vi "Initialization.vi"(8 "error in (no error)":errorcluster, 9 "Side":enum16{"Load", "Drive"}(ring), 10 "CtrlRefs":refnum<vi>[](array[refnum]), 11 "TestSinWaveProc in":refnum<class "TestSinWaveProc.lvclass">) -> (0 "error out":errorcluster, 3 "TestSinWaveProc out":refnum<class "TestSinWaveProc.lvclass">)   [LabVIEW 2024, in "TestSinWaveActor.lvlib" / "TestSinWaveProc.lvclass"]
uses:
  TestSinWaveProc.lvclass
  TestSinWaveProc.lvclass/TestSinWaveProc.ctl
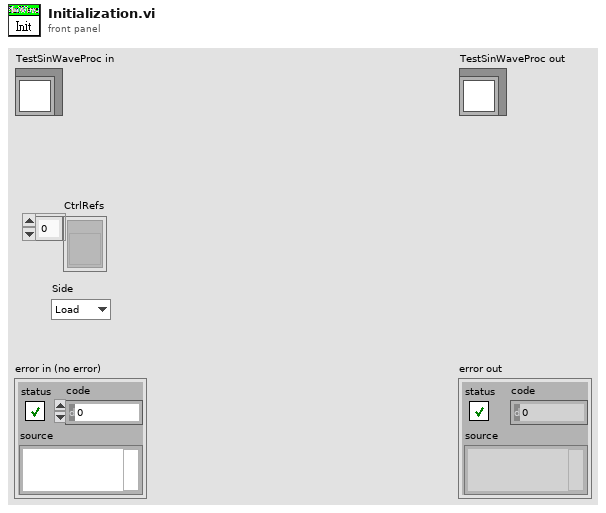
[diagram p1: front panel]
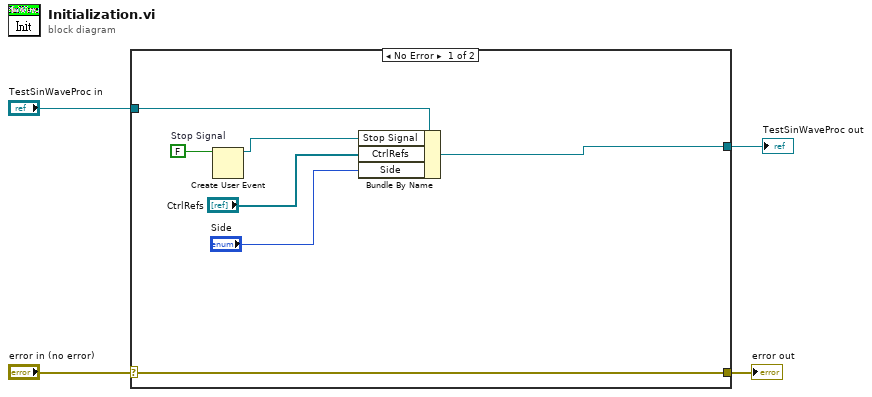
[diagram p0: block diagram]
diagram:
  n1 = case shown="No Error" "error in (no error)" {
    selector: "error in (no error)" -> [w11 w13]
    tunnel: [w11 w13] -> w3
    tunnel: [w6 w12] -> w1
    tunnel: "TestSinWaveProc in" -> [w7 w12]
    frame No Error {
      w10 = FALSE  # Stop Signal
      n2 = Create User Event(user event datatype=w10) -> (user event=w9:refnum<user-event>)  [unwired: 1 in, 1 out]
      n3 = Bundle By Name(cluster=w7, "Stop Signal"=w9, "CtrlRefs"="CtrlRefs", "Side"="Side") -> (w6:refnum<class "TestSinWaveProc.lvclass">)
    }
    frame Error {
    }
  }
  "error out" <- w3
  "TestSinWaveProc out" <- w1
